vi "Read Key.vi"(8 "error in":errorcluster, 10 "Key":string, 11 "E2E configuration in":refnum<class "E2E Tag Exchange configuration.lvclass">) -> (0 "error out":errorcluster, 1 "Value":string, 3 "E2E configuration out":refnum<class "E2E Tag Exchange configuration.lvclass">)   [LabVIEW 2015, in "E2E Tag Exchange configuration.lvclass"]
uses:
  E2E Tag Exchange configuration.lvclass
  E2E Tag Exchange configuration.lvclass/E2E Tag Exchange configuration.ctl
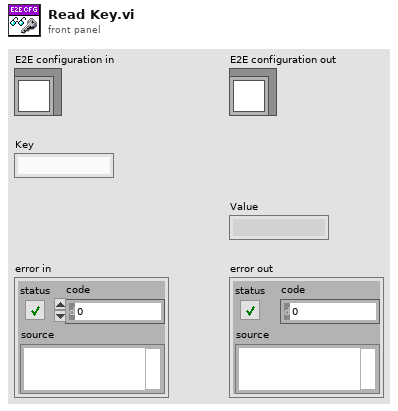
[diagram p1: front panel]
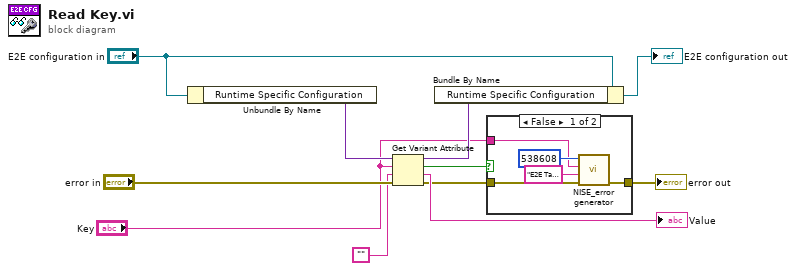
[diagram p0: block diagram]
diagram:
  n1 = Unbundle By Name("E2E configuration in") -> ("Runtime Specific Configuration"=w11:variant)
  n2 = Get Variant Attribute(Variant=w11, name="Key", default value (empty Variant)="", error in="error in") -> (duplicate Variant=w9:variant, found=w4:bool, value=→"Value":string, error out=w3:errorcluster)
  n3 = Bundle By Name(cluster="E2E configuration in", "Runtime Specific Configuration"=w9) -> (→"E2E configuration out":refnum<class "E2E Tag Exchange configuration.lvclass">)
  n4 = case shown="False" w4 {
    tunnel: w3 -> [w16 w17]
    tunnel: [w15 w17] -> w2
    tunnel: "Key" -> [w12 _]
    frame False {
      n5 = call <vilib>:"NISE_error generator.vi"("error in"=w16, "source"="E2E Tag Exchange configuration.lvclass:Read Key.vi", "append error message"=w12, "error code (0)"=538608) -> ("error out"=w15:errorcluster)  [unwired: 5 in]
    }
    frame True {
    }
  }
  "error out" <- w2
